vi "Get path from coef.file (SubVI).vi"(0 "String in":string, 3 "error in":errorcluster) -> (7 "error out":errorcluster)   [LabVIEW 2015]
panel:
  out "path":path
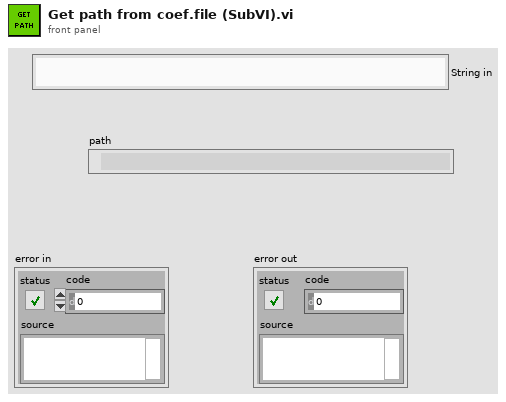
[diagram p1: front panel]
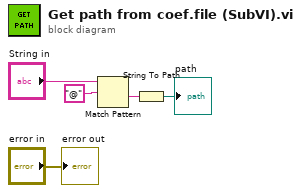
[diagram p0: block diagram]
diagram:
  n1 = Match Pattern(string="String in", regular expression="@") -> (after substring=w3:string)  [unwired: 1 in, 3 out]
  n2 = String To Path(string=w3) -> (path=→"path":path)
  "error out" <- "error in"
